vi "sperren.vi"() -> ()   [LabVIEW 2010]
panel:
  out "Device ID Out":T1(ring)
  in  "Device ID":T1(ring)
  out "error out":errorcluster caption="Fehler (Ausgang)"
  in  "error in (no error)":errorcluster caption="Fehler (Eingang, kein Fehler)"
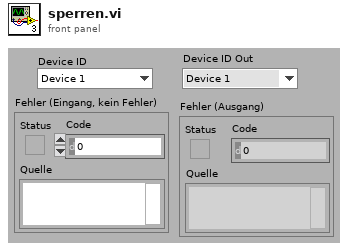
[diagram p1: front panel]
types:
  T1 = enum16{"Device 1", "Device 2", "Device 3", "Device 4", "Device 5", "Device 6", "Device 7", "Device 8"}
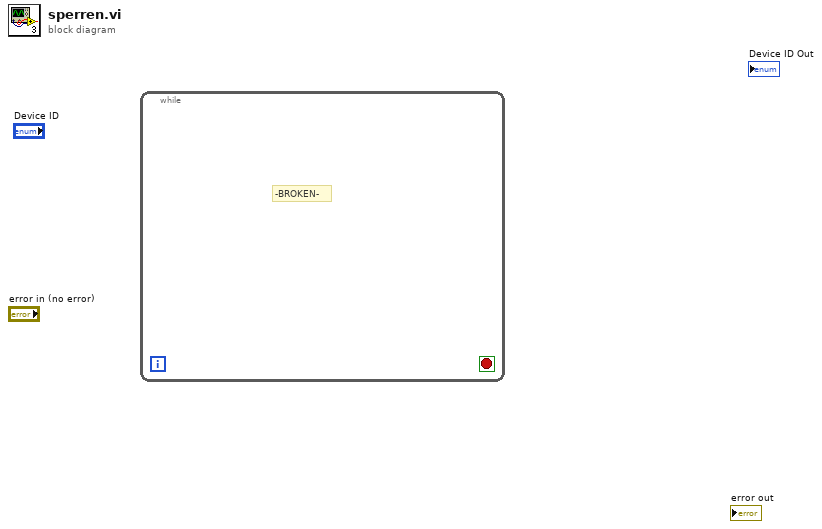
[diagram p0: block diagram]
diagram:
  n1 = while {
    stop <- _ stop-if-true
    # "-BROKEN-"
  }
